vi "Shutdown.vi"(8 "error in (no error)":errorcluster, 11 "Camera_Prime95B in":refnum<class "Camera_Prime95B.lvclass">) -> (0 "error out":errorcluster, 3 "Camera_Prime95B out":refnum<class "Camera_Prime95B.lvclass">)   [LabVIEW 2020, in "Camera_Prime95B.lvlib" / "Camera_Prime95B.lvclass"]
uses:
  Camera_Prime95B.lvclass
  Hardware Abstraction Layer/Component/Device/Device/DeviceStatus.ctl
  Camera_Prime95B.lvclass/Camera_Prime95B.ctl
  E:/Development/DevHardSoftware/MicroscopyFramework/Model/Hardware Layer/Real Hardware/Camera_Prime95B/Camera_Prime95B/Dependencies/PVCamNET.dll
  Dependencies/PVCamNET.dll
  Hardware Abstraction Layer/Component/Camera/Camera/Camera.lvclass
  Hardware Abstraction Layer/Component/Device/Device/Device.lvlib
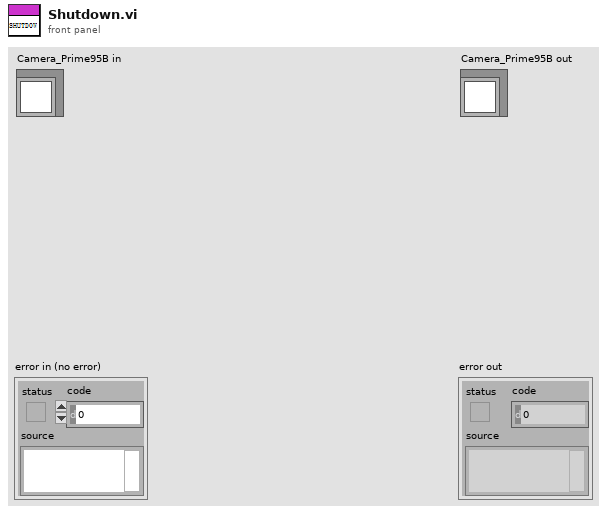
[diagram p1: front panel]
types:
  T1 = typedef "Device.lvlib/DeviceStatus.ctl" = i32
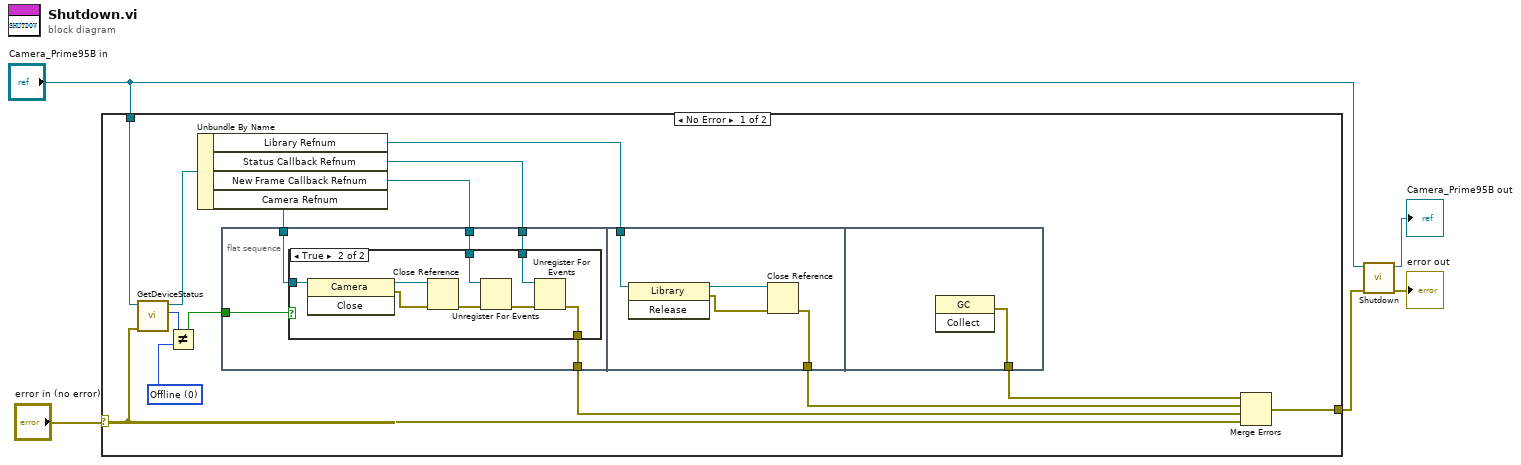
[diagram p0: block diagram]
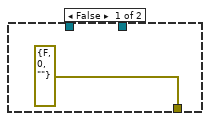
[diagram p2: hidden frame]
diagram:
  n1 = case shown="No Error" "error in (no error)" {
    selector: "error in (no error)" -> [w12 w39]
    tunnel: [w17 w39] -> w2
    tunnel: "Camera_Prime95B in" -> [w19 _]
    frame No Error {
      w10 = T1 0 items=["Offline", "Idle", "Busy"] ("y")
      n2 = call-dynamic "GetDeviceStatus.vi"("error in (no error)"=w12, "Camera_Prime95B in"=w19) -> ("Status"=w11:T1, "Camera_Prime95B out"=w13:refnum<class "Camera_Prime95B.lvclass">)  [unwired: 7 in, 1 out]
      n3 = Not Equal?(x=w11, y=w10) -> (x != y?=w9:bool)
      n4 = Unbundle By Name(w13) -> ("Library Refnum"=w8:refnum<k24>, "Status Callback Refnum"=w6:refnum<k27>, "New Frame Callback Refnum"=w7:refnum<k27>, "Camera Refnum"=w18:refnum<k24>)
      n5 = flat-sequence {
        tunnel: w18 -> [w24]
        tunnel: [w23] -> w16
        tunnel: w9 -> [w22]
        tunnel: w7 -> [w21]
        tunnel: w6 -> [w20]
        tunnel: [w35] -> w15
        tunnel: w8 -> [w34]
        tunnel: [w38] -> w14
        frame #0 {
          n6 = case shown="True" w22 {
            tunnel: w24 -> [_ w33]
            tunnel: [errorcluster {"status"=FALSE, "code"=0, "source"=""} ("error out") w26] -> w23
            tunnel: w21 -> [_ w28]
            tunnel: w20 -> [_ w27]
            frame False {
            }
            frame True {
              n7 = invoke class="Camera" method="Close"(reference=w33) -> (reference out=w32:refnum<k24>, error out=w31:errorcluster)  [unwired: 2 in, 1 out]
              n8 = Close Reference(reference=w32, error in (no error)=w31) -> (error out=w29:errorcluster)
              n9 = Unregister For Events(event registration refnum=w28, error in=w29) -> (error out=w30:errorcluster)
              n10 = Unregister For Events(event registration refnum=w27, error in=w30) -> (error out=w26:errorcluster)
            }
          }
        }
        frame #1 {
          n11 = invoke class="Library" method="Release"(reference=w34) -> (reference out=w36:refnum<k24>, error out=w37:errorcluster)  [unwired: 2 in, 1 out]
          n12 = Close Reference(reference=w36, error in (no error)=w37) -> (error out=w35:errorcluster)
        }
        frame #2 {
          n13 = invoke class="GC" method="Collect"() -> (error out=w38:errorcluster)  [unwired: 3 in, 2 out]
        }
      }
      n14 = Merge Errors(w14, w15, w16, w12) -> (w17:errorcluster)
    }
    frame Error {
    }
  }
  n15 = call-parent "Shutdown.vi"("error in (no error)"=w2, "Device in"="Camera_Prime95B in") -> ("error out"=→"error out":errorcluster, "Device out"=→"Camera_Prime95B out":refnum<class "Camera_Prime95B.lvclass">)  [unwired: 8 in]
